vi "PlanificationScenarios.vi"() -> (5 "Canceled?":bool)   [LabVIEW 2015]
uses:
  scan_array.llb/Scan Array (I32).vi
  <vilib>/httpClient/LabVIEWHTTPClient.lvlib
panel:
  out "element":string
  in  "String 3":string
  in  "String 2":string
  in  "String":string
  out "body 2":string
  out "body":string
  in  "OK Button 2":bool
  out "subarray":string[](array[string])
  in  "Combo Box 2":string(combo)
  in  "Combo Box":string(combo)
  in  "OK":bool
  in  "All":bool
  in  "List":i32(listbox)
  # "Donner date de scénario"
  # "Choisir scénario"
  # "Choisir une chambre"
  # "Donner heure de début"
  # "Donner heure de fin"
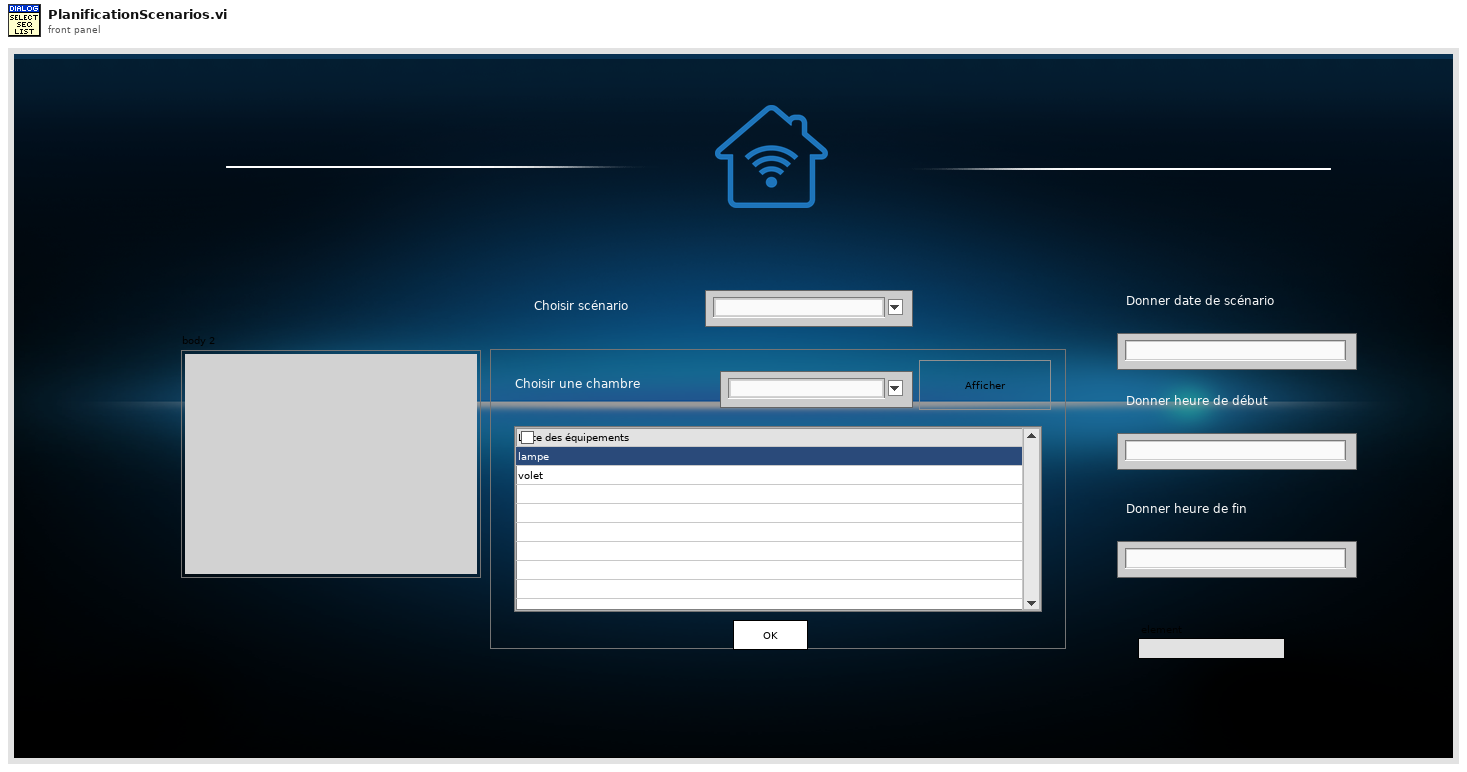
[diagram p1: front panel]
types:
  T1 = enum32{"Invalid", "Standard", "Closed", "Hidden", "Minimized", "Maximized"}
  T2 = typedef "LVPoint32TypeDef.ctl" = cluster{"Horizontal":i32, "Vertical":i32}
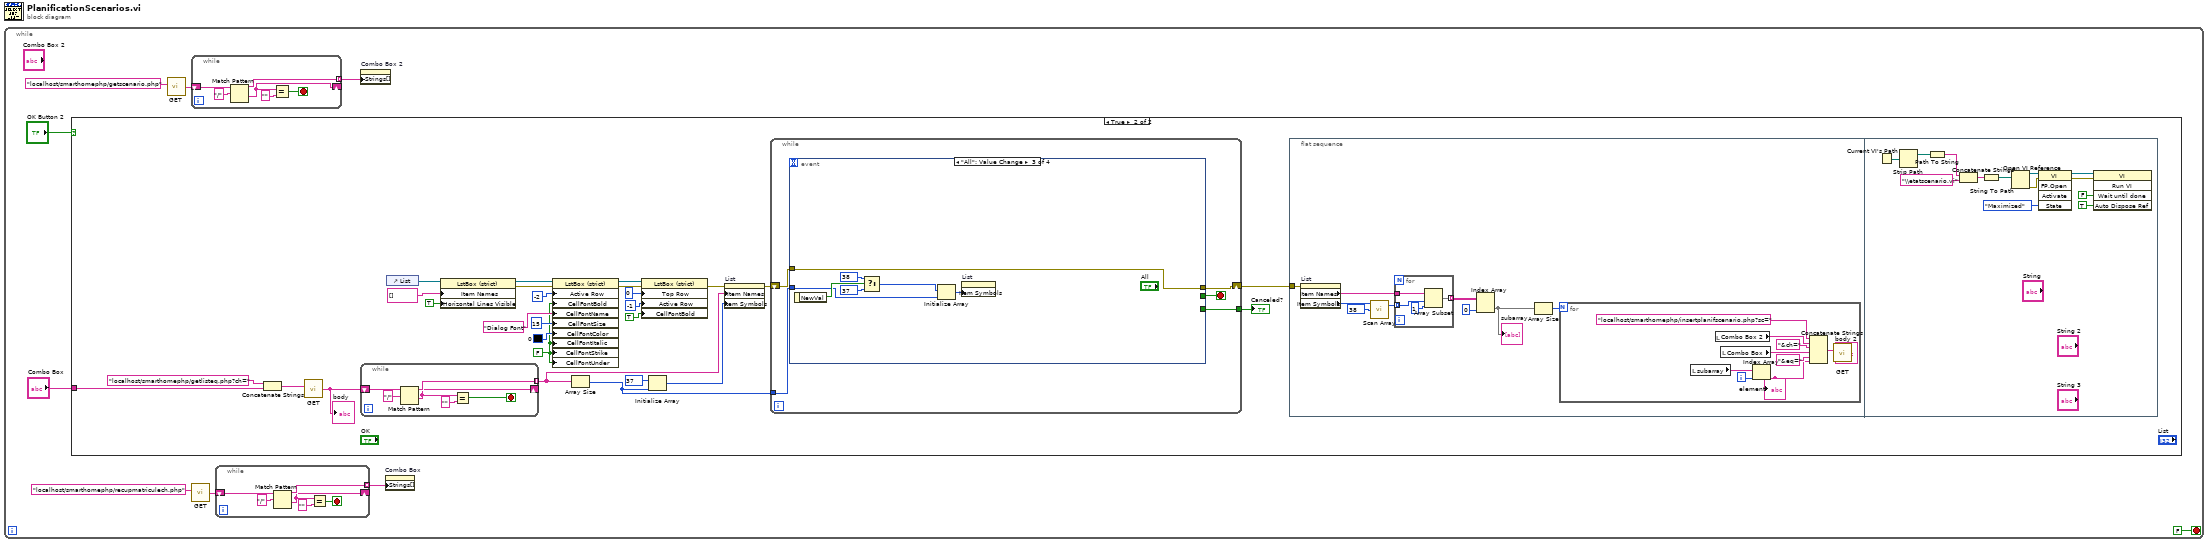
[diagram p0: block diagram]
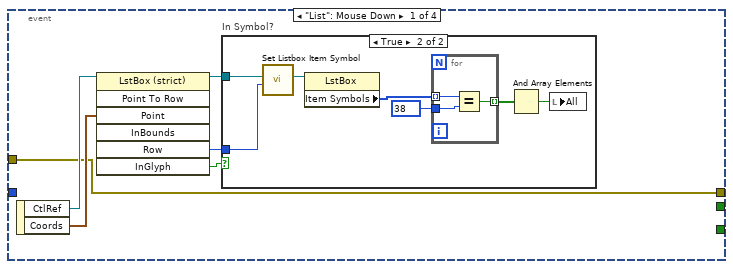
[diagram p3: hidden frame]
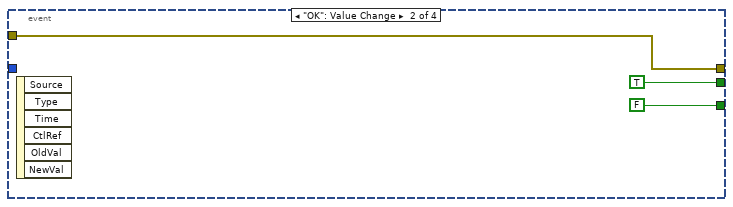
[diagram p5: hidden frame]
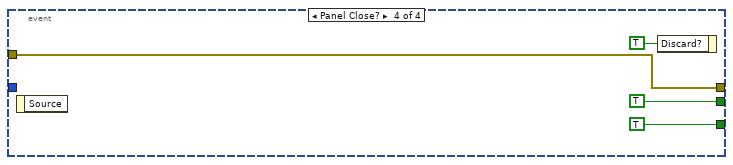
[diagram p6: hidden frame]
diagram:
  n1 = while {
    stop <- FALSE stop-if-true
    n2 = case shown="True" "OK Button 2" {
      tunnel: "Combo Box" -> [_ w13]
      frame False {
      }
      frame True {
        w22 = FALSE ("Active Row:Cell Font:Bold")
        n3 = Concatenate Strings("localhost/smarthomephp/getlisteq.php?ch=", w13) -> (w12:string)
        n4 = call <vilib>:"GET.vi"("url"=w12) -> ("body"=w11:string)  [unwired: 11 in, 3 out]
        "body" <- w11
        n5 = while {
          tunnel: [w76] -> w10 mode=indexing
          shift-right: [w73] -> _
          shift-left: w11 -> [w78]
          stop <- w74 stop-if-true
          n6 = Match Pattern(string=w78, regular expression="/") -> (before substring=w76:string, after substring=w73:string)  [unwired: 1 in, 2 out]
          n7 = Equal?(x=w73, y="") -> (x = y?=w74:bool)
        }
        n8 = control-ref of="List"() -> (w20:refnum<vi>)
        n9 = property class="LstBox (strict)"(reference=w20, "Item Names"=string[] [], "Horizontal Lines Visible"=TRUE ("Visible Items:Horizontal Lines Visible")) -> (reference out=w28:refnum<vi>, error out=w26:errorcluster)  [unwired: 1 in]
        n10 = property on="Property Node" class="LstBox (strict)"(reference=w28, error in=w26, "Active Row"=-2 ("Active Row:Active Row Number"), "CellFontBold"=w22, "CellFontName"="Dialog Font" ("Active Row:Cell Font:Name"), "CellFontSize"=u32 15 ("Active Row:Cell Font:Size"), "CellFontColor"=u32 0, "CellFontItalic"=w22, "CellFontStrike"=w22, "CellFontUnder"=w22) -> (reference out=w17:refnum<vi>, error out=w18:errorcluster)
        n11 = Array Size(array=w10) -> (size(s)=w32:i32)
        n12 = property class="LstBox (strict)"(reference=w17, error in=w18, "Top Row"=0, "Active Row"=-1 ("Active Row:Active Row Number"), "CellFontBold"=TRUE ("Active Row:Cell Font:Bold")) -> (error out=w16:errorcluster)  [unwired: 1 out]
        n13 = Initialize Array(37, w32) -> (w35:i32[])
        n14 = property on="List" class="LstBox (strict)"(error in=w16, "Item Names"=w10, "Item Symbols"=w35) -> (error out=w15:errorcluster)  [unwired: 1 in, 1 out]
        n15 = while {
          shift-right: [w82] -> w34
          shift-left: w15 -> [w83]
          tunnel: [w80] -> w33
          tunnel: w32 -> [w79]
          stop <- w81 stop-if-true
          n16 = event shown="[2] \"All\": Value Change" {
            selector: _ -> [_ _ _ _]
            dyn-events: _ -> [_ _ _ _]
            timeout: _ -> [_ _ _ _]
            tunnel: w83 -> [w84 w101 w103 w112]
            tunnel: [w84 w101 w103 w112] -> w82
            tunnel: [_ TRUE ("NewVal") _ TRUE ("NewVal")] -> w81
            tunnel: [_ FALSE _ TRUE] -> w80
            tunnel: w79 -> [_ _ w105 _]
            event "List": Mouse Down {
              n17 = event-data() -> ("CtlRef"=w89:refnum<vi>, "Coords"=w86:T2)  [unwired: 1 in]
              n18 = invoke class="LstBox (strict)" method="Point To Row"(reference=w89, "Point"=w86) -> (reference out=w85:refnum<vi>, "Row"=w87:i32, "InGlyph"=w88:bool)  [unwired: 5 in, 4 out]
              n19 = case "In Symbol?" shown="True" w88 {
                tunnel: w87 -> [_ w95]
                tunnel: w85 -> [_ w96]
                frame False {
                }
                frame True {
                  n20 = call "Set Listbox Item Symbol.vi"("Row"=w95, "Listbox"=w96) -> ("dup Listboc"=w94:refnum<vi>)  [unwired: 6 in]
                  n21 = property class="LstBox"(reference=w94) -> ("Item Symbols"=w93:i32[])  [unwired: 1 in, 2 out]
                  n22 = for {
                    tunnel: w93 -> [w99] mode=indexing
                    tunnel: 38 -> [w98]
                    tunnel: [w97] -> w91 mode=indexing
                    n23 = Equal?(x=w99, y=w98) -> (x = y?=w97:bool)
                  }
                  n24 = And Array Elements(Boolean array=w91) -> (logical AND=w90:bool)
                  n25 = local write "All"(w90) -> ()
                }
              }
            }
            event "OK": Value Change {
              n26 = event-data() -> ()  [unwired: 1 in, 6 out]
            }
            event "All": Value Change {
              n27 = event-data() -> ("NewVal"=w109:bool)  [unwired: 1 in]
              n28 = Select(t=38, s=w109, f=37) -> (s? t:f=w106:i32)
              n29 = Initialize Array(w106, w105) -> (w104:i32[])
              n30 = property on="List" class="LstBox (strict)"("Item Symbols"=w104) -> ()  [unwired: 2 in, 2 out]
            }
            event Panel Close? {
              n31 = event-data() -> ()  [unwired: 1 in, 1 out]
              n32 = event-data("Discard?"=TRUE) -> ()  [unwired: 1 in, 1 out]
            }
          }
        }
        "Canceled?" <- w33
        n33 = flat-sequence {
          tunnel: w34 -> [w45]
          frame #0 {
            n34 = property on="List" class="LstBox (strict)"(error in=w45) -> ("Item Names"=w39:string[], "Item Symbols"=w43:i32[])  [unwired: 1 in, 2 out]
            n35 = call-poly "Scan Array.vi"("search element"=38, "Input array"=w43) -> ("Matched Indices"=w42:i32[])  [unwired: 3 in]
            n36 = for {
              tunnel: w42 -> [w59] mode=indexing
              tunnel: [w57] -> w41 mode=indexing
              tunnel: w39 -> [w56]
              n37 = Array Subset(array=w56, index=w59, length=1) -> (w57:string[])
            }
            n38 = Index Array(array=w41, index (col)=0 ("index (row)")) -> (element=w38:string[])  [unwired: 1 in]
            "subarray" <- w38
            n39 = Array Size(array=w38) -> (size(s)=w37:i32)
            n40 = for {
              N: w37 -> [_]
              i -> [w55]
              n41 = local read "subarray"() -> (w54:string[])
              n42 = local read "Combo Box 2"() -> (w52:string)
              n43 = local read "Combo Box"() -> (w50:string)
              n44 = Index Array(array=w54, index=w55) -> (element=w48:string)
              "element" <- w48
              n45 = Concatenate Strings("localhost/smarthomephp/insertplanifscenario.php?sc=", w52, "&ch=", w50, "&eq=", w48) -> (w47:string)
              n46 = call <vilib>:"GET.vi"("url"=w47) -> ("body"=→"body 2":string)  [unwired: 11 in, 3 out]
            }
          }
          frame #1 {
            n47 = Current VI's Path() -> (path=w72:path)
            n48 = Strip Path(path=w72) -> (stripped path=w71:path)  [unwired: 1 out]
            n49 = Path To String(path=w71) -> (string=w70:string)
            n50 = Concatenate Strings(w70, "\\etatscenario.vi") -> (w68:string)
            n51 = String To Path(string=w68) -> (path=w67:path)
            n52 = Open VI Reference(vi path=w67) -> (vi reference=w66:refnum<vi>, error out=w65:errorcluster)  [unwired: 5 in]
            n53 = invoke class="VI" method="FP.Open"(reference=w66, error in=w65, "State"=T1."Maximized") -> (reference out=w64:refnum<vi>, error out=w63:errorcluster)  [unwired: 2 in, 3 out]
            n54 = invoke class="VI" method="Run VI"(reference=w64, error in=w63, "Wait until done"=FALSE ("Wait Until Done"), "Auto Dispose Ref"=TRUE ("Auto Dispose Reference")) -> ()  [unwired: 1 in, 5 out]
          }
        }
      }
    }
    n55 = call <vilib>:"GET.vi"("url"="localhost/smarthomephp/getscenario.php") -> ("body"=w8:string)  [unwired: 11 in, 3 out]
    n56 = while {
      tunnel: [w123] -> w7 mode=indexing
      shift-right: [w120] -> _
      shift-left: w8 -> [w125]
      stop <- w121 stop-if-true
      n57 = Match Pattern(string=w125, regular expression="/") -> (before substring=w123:string, after substring=w120:string)  [unwired: 1 in, 2 out]
      n58 = Equal?(x=w120, y="") -> (x = y?=w121:bool)
    }
    n59 = call <vilib>:"GET.vi"("url"="localhost/smarthomephp/recupmatriculech.php") -> ("body"=w6:string)  [unwired: 11 in, 3 out]
    n60 = while {
      tunnel: [w117] -> w4 mode=indexing
      shift-right: [w114] -> _
      shift-left: w6 -> [w119]
      stop <- w115 stop-if-true
      n61 = Match Pattern(string=w119, regular expression="/") -> (before substring=w117:string, after substring=w114:string)  [unwired: 1 in, 2 out]
      n62 = Equal?(x=w114, y="") -> (x = y?=w115:bool)
    }
    n63 = property on="Combo Box 2" class="CmbBox"("Strings[]"=w7) -> ()  [unwired: 2 in, 2 out]
    n64 = property on="Combo Box" class="CmbBox"("Strings[]"=w4) -> ()  [unwired: 2 in, 2 out]
  }
